vi "Build Project PPL.vi"(0 "LVLIB Path":path, 1 "Exclude dependent packed libraries":bool=TRUE, 2 "Exclusions":T1={"Disconnect type definitions"=FALSE, "Remove unused polymorphic VI instances"=TRUE, "Remove unused members of project libraries"=TRUE, "Modify project library file after removing unused members"=TRUE}, 3 "Always Included Files":path[](array[path]), 5 "Build Name":string, 9 "Proj Ref":refnum<vi>, 11 "error in (no error)":errorcluster, 12 "PPL Dir":path, 14 "Version number":T2) -> (4 "GeneratedFiles":path[](array[path]), 6 "LVLIB Path Out":path, 10 "Proj Ref Out":refnum<vi>, 15 "error out":errorcluster)   [LabVIEW 2018]
uses:
  <vilib>/AppBuilder/AB_API/common/AB_API Version Number.ctl
  <vilib>/AppBuilder/AB_API/common/AB_API Primary Exclusions.ctl
  <vilib>/AppBuilder/AB_API/common/AB_API Default Destinations.ctl
  <vilib>/AppBuilder/AB_API/PPL/NI_AB_API_PPL.lvclass
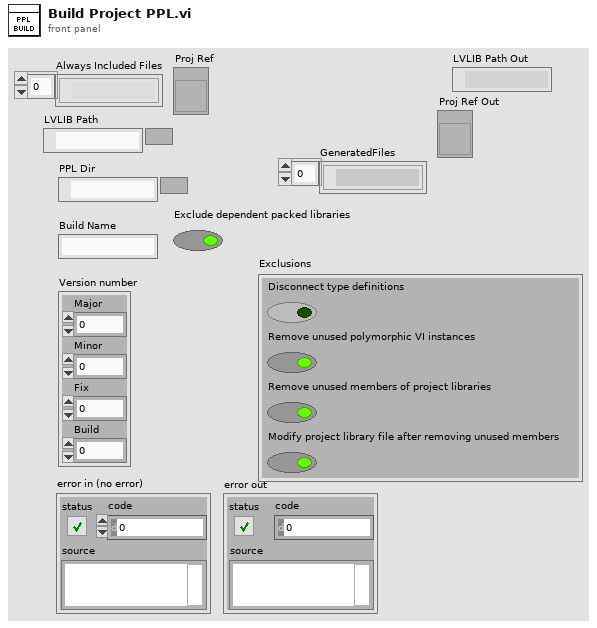
[diagram p1: front panel]
types:
  T1 = typedef "AB_API Primary Exclusions.ctl" = cluster{"Disconnect type definitions":bool, "Remove unused polymorphic VI instances":bool, "Remove unused members of project libraries":bool, "Modify project library file after removing unused members":bool}
  T2 = typedef "AB_API Version Number.ctl" = cluster{"Major":u16, "Minor":u16, "Fix":u16, "Build":u16}
  T3 = typedef "AB_API Default Destinations.ctl" = enum16{"Destination Directory", "Support Directory"}
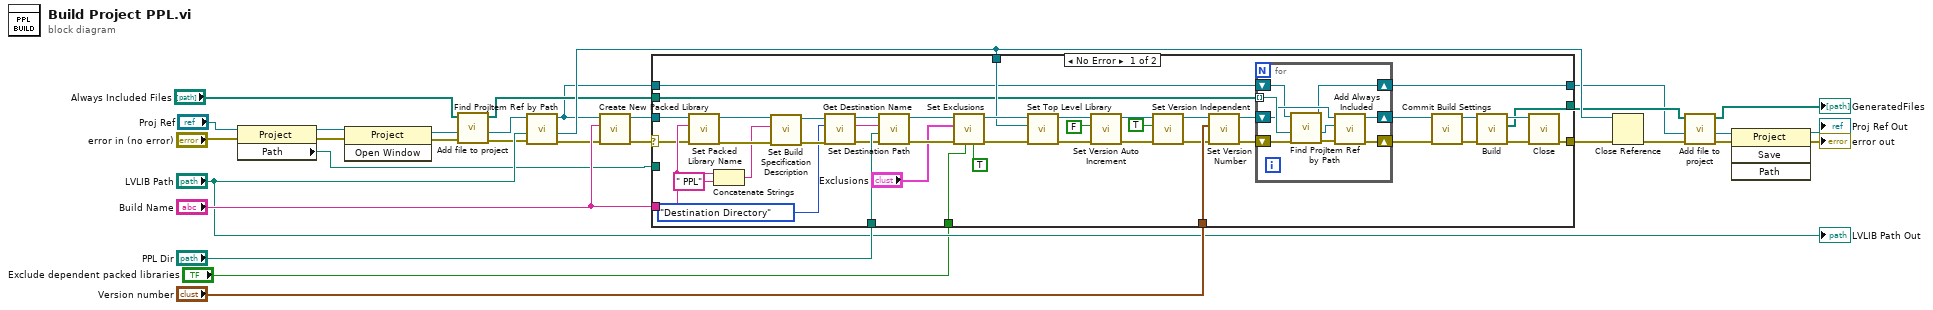
[diagram p0: block diagram]
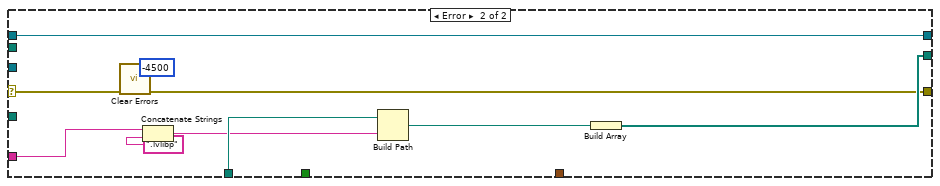
[diagram p2: hidden frame]
diagram:
  n1 = property class="Project"(reference="Proj Ref", error in="error in (no error)") -> (reference out=w14:refnum<vi>, error out=w13:errorcluster, "Path"=w12:path)
  n2 = invoke class="Project" method="Open Window"(reference=w14, error in=w13) -> (reference out=w8:refnum<vi>, error out=w9:errorcluster)  [unwired: 1 in, 1 out]
  n3 = call "Add file to project.vi"("error in"=w9, "Project Ref in"=w8, "File Path"="Always Included Files") -> ("error out"=w6:errorcluster, "Project out"=w5:refnum<vi>, "Actual File Path"=w4:path[])  [unwired: 6 in]
  n4 = call "Find ProjItem Ref by Path.vi"("error in (no error)"=w6, "Path"="LVLIB Path", "Proj Ref In"=w5) -> ("error out"=w26:errorcluster, "ProjectItem Refnum"=w24:refnum<vi>, "Proj Ref Out"=w3:refnum<vi>)  [unwired: 6 in]
  n5 = call <vilib>:"Create New Packed Library.vi"("error in (no error)"=w26, "Build specification name"="Build Name", "Project Refnum"=w3) -> ("error out"=w18:errorcluster, "PPL out"=w27:refnum<class "NI_AB_API_PPL.lvclass">)  [unwired: 7 in]
  n6 = case shown="No Error" w18 {
    selector: w18 -> [w45 w93]
    tunnel: "Version number" -> [w74 _]
    tunnel: "PPL Dir" -> [w73 w91]
    tunnel: "Build Name" -> [w72 w90]
    tunnel: [w71 w87] -> w17
    tunnel: w27 -> [w69 _]
    tunnel: w24 -> [w47 _]
    tunnel: [w46 w88] -> w22
    tunnel: w12 -> [_ _]
    tunnel: w4 -> [w40 _]
    tunnel: w3 -> [w39 w84]
    tunnel: [w38 w84] -> w2
    tunnel: "Exclude dependent packed libraries" -> [w36 _]
    frame No Error {
      n7 = call-dynamic "Set Packed Library Name.vi"("error in (no error)"=w45, "Packed library name"=w72, "PPL in"=w69) -> ("error out"=w68:errorcluster, "PPL out"=w67:refnum<class "NI_AB_API_PPL.lvclass">)  [unwired: 7 in]
      n8 = Concatenate Strings(w72, " PPL" ("string")) -> (w58:string)
      n9 = call-dynamic "Set Build Specification Description.vi"("error in (no error)"=w68, "Build Specification Description"=w58, "NI_AB_API_PPL in"=w67) -> ("error out"=w66:errorcluster, "NI_AB_API_PPL out"=w70:refnum<class "NI_AB_API_PPL.lvclass">)  [unwired: 7 in]
      n10 = call-dynamic "Get Destination Name.vi"("error in (no error)"=w66, "Default Destinations"=AB_API_Default_Destinations."Destination Directory", "PPL in"=w70) -> ("error out"=w62:errorcluster, "Destination Name"=w64:string, "PPL out"=w63:refnum<class "NI_AB_API_PPL.lvclass">)  [unwired: 6 in]
      n11 = call-dynamic "Set Destination Path.vi"("error in (no error)"=w62, "Destination path"=w73, "Destination label"=w64, "PPL in"=w63) -> ("error out"=w59:errorcluster, "PPL out"=w60:refnum<class "NI_AB_API_PPL.lvclass">)  [unwired: 6 in]
      n12 = call-dynamic "Set Exclusions.vi"("Exclude dependent shared libraries"=TRUE ("Exclude dependent packed libraries"), "Exclude dependent packed libraries"=w36, "error in (no error)"=w59, "Exclusions"="Exclusions", "PPL in"=w60) -> ("error out"=w56:errorcluster, "PPL out"=w55:refnum<class "NI_AB_API_PPL.lvclass">)  [unwired: 5 in]
      n13 = call-dynamic "Set Top Level Library.vi"("error in (no error)"=w56, "ProjectItem Refnum"=w47, "PPL in"=w55) -> ("error out"=w54:errorcluster, "PPL out"=w52:refnum<class "NI_AB_API_PPL.lvclass">)  [unwired: 7 in]
      n14 = call-dynamic "Set Version Auto Increment.vi"("error in (no error)"=w54, "Auto Increment Version"=FALSE, "NI_AB_API_PPL in"=w52) -> ("error out"=w35:errorcluster, "NI_AB_API_PPL out"=w32:refnum<class "NI_AB_API_PPL.lvclass">)  [unwired: 7 in]
      n15 = call-dynamic "Set Version Independent.vi"("error in (no error)"=w35, "versionIndependent"=TRUE, "NI_AB_API_PPL in"=w32) -> ("error out"=w34:errorcluster, "NI_AB_API_PPL out"=w33:refnum<class "NI_AB_API_PPL.lvclass">)  [unwired: 7 in]
      n16 = call-dynamic "Set Version Number.vi"("error in (no error)"=w34, "Version number"=w74, "PPL in"=w33) -> ("error out"=w44:errorcluster, "PPL out"=w43:refnum<class "NI_AB_API_PPL.lvclass">)  [unwired: 7 in]
      n17 = for {
        shift-right: [w83] -> w42
        shift-left: w44 -> [w81]
        shift-right: [w82] -> w41
        shift-left: w43 -> [w77]
        tunnel: w40 -> [w79] mode=indexing
        shift-right: [w75] -> w38
        shift-left: w39 -> [w76]
        n18 = call "Find ProjItem Ref by Path.vi"("error in (no error)"=w81, "Path"=w79, "Proj Ref In"=w76) -> ("error out"=w80:errorcluster, "ProjectItem Refnum"=w78:refnum<vi>, "Proj Ref Out"=w75:refnum<vi>)  [unwired: 6 in]
        n19 = call-dynamic "Add Always Included.vi"("error in (no error)"=w80, "ProjectItem Refnum"=w78, "PPL in"=w77) -> ("error out"=w83:errorcluster, "PPL out"=w82:refnum<class "NI_AB_API_PPL.lvclass">)  [unwired: 7 in]
      }
      n20 = call-dynamic "Commit Build Settings.vi"("error in (no error)"=w42, "PPL in"=w41) -> ("error out"=w48:errorcluster, "PPL out"=w50:refnum<class "NI_AB_API_PPL.lvclass">)  [unwired: 8 in]
      n21 = call-dynamic "Build.vi"("error in (no error)"=w48, "PPL in"=w50) -> ("error out"=w49:errorcluster, "GeneratedFiles"=w46:path[], "PPL out"=w51:refnum<class "NI_AB_API_PPL.lvclass">)  [unwired: 6 in, 1 out]
      n22 = call-dynamic "Close.vi"("error in (no error)"=w49, "DLL in"=w51) -> ("error out"=w71:errorcluster)  [unwired: 9 in]
    }
    frame Error {
      n23 = call <vilib>:"Clear Errors.vi"("error in (no error)"=w93, "specific error code to clear (0: all)"=-4500) -> ("error out"=w87:errorcluster)  [unwired: 4 in, 1 out]
      n24 = Concatenate Strings(w90, ".lvlibp") -> (w85:string)
      n25 = Build Path(base path=w91, name or relative path=w85) -> (appended path=w86:path)
      n26 = Build Array(w86) -> (w88:path[])
    }
  }
  n27 = Close Reference(reference=w24, error in (no error)=w17) -> (error out=w23:errorcluster)
  n28 = call "Add file to project.vi"("error in"=w23, "Project Ref in"=w2, "File Path"=w22) -> ("error out"=w20:errorcluster, "Project out"=w21:refnum<vi>, "Actual File Path"=→"GeneratedFiles":path[])  [unwired: 6 in]
  n29 = invoke class="Project" method="Save"(reference=w21, error in=w20) -> (reference out=→"Proj Ref Out":refnum<vi>, error out=→"error out":errorcluster)  [unwired: 2 in, 2 out]
  "LVLIB Path Out" <- "LVLIB Path"
